vi "AIT 429 - Clear Database.vi"(8 "error in (no error)":errorcluster, 11 "Node Ptr":u64 format="%.0x") -> (0 "error out":errorcluster)   [LabVIEW 2015, in "AIT 429 System Explorer.lvlib"]
uses:
  Shared/Controls and Global/Global.vi
  <vilib>/NI Veristand/Custom Device Tools/Custom Device Utility Library/NI VeriStand - Search for Item by GUID.vi
  AIT 429 System Explorer.lvlib
  <vilib>/NI Veristand/Custom Device API/Custom Device API.lvlib
  Shared/AIT 429 Shared.lvlib
  <vilib>/NI Veristand/Custom Device Tools/Custom Device Utility Library/Custom Device Utility Library.lvlib
panel:
  in  "Tag":string
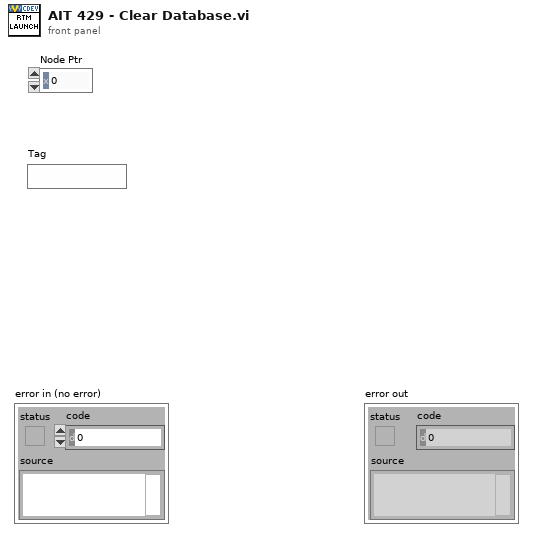
[diagram p1: front panel]
types:
  T1 = typedef "Custom Device API.lvlib/Custom Device Item Ref.ctl" = u64
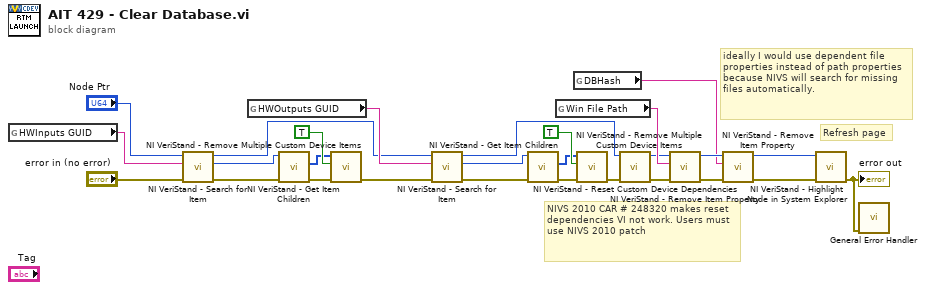
[diagram p0: block diagram]
diagram:
  # "ideally I would use dependent file properties instead of path properties because NIVS will search for missing files automatically."
  # "NIVS 2010 CAR # 248320 makes reset dependencies VI not work. Users must use NIVS 2010 patch"
  # "Refresh page"
  n1 = global read "Global.vi" "HWInputs GUID"() -> (w20:string)
  n2 = call-poly <vilib>:"NI VeriStand - Search for Item.vi"("error in"="error in (no error)", "Item GUID"=w20, "Section Ref in"="Node Ptr") -> ("error out"=w15:errorcluster, "Item Ref"=w18:T1, "Section Ref out"=w8:T1)  [unwired: 5 in, 1 out]
  n3 = global read "Global.vi" "HWOutputs GUID"() -> (w13:string)
  n4 = call <vilib>:"NI VeriStand - Get Item Children.vi"("error in (no error)"=w15, "Item Ref in"=w18) -> ("error out"=w27:errorcluster, "Child Refs"=w22:T1[])  [unwired: 6 in, 2 out]
  n5 = call <vilib>:"NI VeriStand - Remove Multiple Custom Device Items.vi"("error in (no error)"=w27, "Force Delete (F)"=TRUE, "Item Refs in"=w22) -> ("error out"=w14:errorcluster)  [unwired: 7 in, 1 out]
  n6 = call-poly <vilib>:"NI VeriStand - Search for Item.vi"("error in"=w14, "Item GUID"=w13, "Section Ref in"=w8) -> ("error out"=w11:errorcluster, "Item Ref"=w12:T1, "Section Ref out"=w7:T1)  [unwired: 5 in, 1 out]
  n7 = call <vilib>:"NI VeriStand - Get Item Children.vi"("error in (no error)"=w11, "Item Ref in"=w12) -> ("error out"=w16:errorcluster, "Child Refs"=w10:T1[])  [unwired: 6 in, 2 out]
  n8 = global read "Global.vi" "Win File Path"() -> (w24:string)
  n9 = global read "Global.vi" "DBHash"() -> (w1:string)
  n10 = call <vilib>:"NI VeriStand - Remove Multiple Custom Device Items.vi"("error in (no error)"=w16, "Force Delete (F)"=TRUE, "Item Refs in"=w10) -> ("error out"=w9:errorcluster)  [unwired: 7 in, 1 out]
  n11 = call <vilib>:"NI VeriStand - Reset Custom Device Dependencies.vi"("error in (no error)"=w9, "Device Ref in"=w7) -> ("error out"=w25:errorcluster, "Device Ref out"=w23:T1)  [unwired: 8 in]
  n12 = call <vilib>:"NI VeriStand - Remove Item Property.vi"("error in (no error)"=w25, "Property Name"=w24, "Item Ref in"=w23) -> ("error out"=w5:errorcluster, "Item Ref out"=w4:T1)  [unwired: 6 in, 1 out]
  n13 = call <vilib>:"NI VeriStand - Remove Item Property.vi"("error in (no error)"=w5, "Property Name"=w1, "Item Ref in"=w4) -> ("error out"=w3:errorcluster, "Item Ref out"=w2:T1)  [unwired: 6 in, 1 out]
  n14 = call <vilib>:"NI VeriStand - Highlight Node in System Explorer.vi"("error in (no error)"=w3, "Item Ref in"=w2) -> ("error out"=w6:errorcluster)  [unwired: 8 in, 1 out]
  "error out" <- w6
  n15 = call <vilib>:"General Error Handler.vi"("error in (no error)"=w6) -> ()  [unwired: 10 in, 5 out]
